vi "emi_Error State Changed(no error Init).vi"(9 "Error Inn":errorcluster) -> (3 "Changed and Is Error Or Warning":bool, 6 "changed and Is Error":bool, 8 "changed":bool, 10 "error out":errorcluster)   [LabVIEW 2010]
doc: "Monitors an Error State, indicateing change. \n\nFirst call will give false if no error, and true if error. (Note, unlike other change monitors in this library)\n\nreentrant Subroutine."
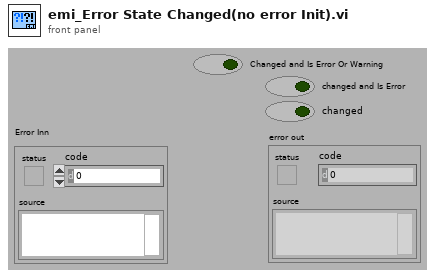
[diagram p1: front panel]
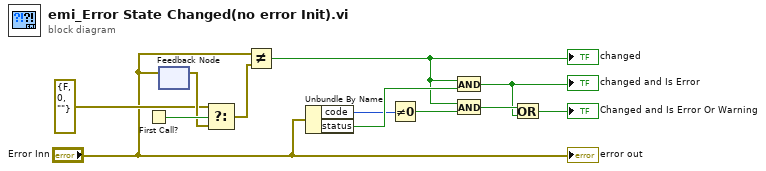
[diagram p0: block diagram]
diagram:
  n1 = First Call?() -> (First Call?: T/F=w12:bool)
  n2 = feedback-in #1("Error Inn") -> ()
  n3 = feedback #1() -> (w11:errorcluster)  [unwired: 1 in]
  n4 = Select(t=errorcluster {"status"=FALSE, "code"=0, "source"=""}, s=w12, f=w11) -> (s? t:f=w10:errorcluster)
  n5 = Not Equal?(x="Error Inn", y=w10) -> (x != y?=w1:bool)
  "changed" <- w1
  n6 = Unbundle By Name("Error Inn") -> ("code"=w7:i32, "status"=w8:bool)
  n7 = Not Equal To 0?(x=w7) -> (x != 0?=w6:bool)
  n8 = And(x=w1, y=w8) -> (x .and. y?=w4:bool)
  "changed and Is Error" <- w4
  n9 = And(x=w1, y=w6) -> (x .and. y?=w5:bool)
  n10 = Or(x=w5, y=w4) -> (x .or. y?=→"Changed and Is Error Or Warning":bool)
  "error out" <- "Error Inn"
